vi "main.vi"() -> ()   [LabVIEW 2018]
uses:
  Interface/Interface.lvclass
  Interface/Interface.lvclass/Interface.ctl
  CCD/CCD.lvclass/CCD.ctl
  Timer/Timer.lvclass/Timer.ctl
  JSON/JSON.lvclass/JSON.ctl
  CCD/CCD.lvclass
  Timer/Timer.lvclass
  JSON/JSON.lvclass
  State Machine/State Machine.lvclass
  Cooler/Cooler.lvclass
panel:
  in  "Camera Setup":T1={"Exposure Time"=1e-05, "Readout Rate"=0, "Pre-amp gain"=0, "Initial Line"=1, "Final Line"=1024, "Final Column"=1024, "Initial Cloumn"=1, "Binning"=1, "EM Gain"=2, "EM Mode"=0, "Kinetic Series Length"=1} {"Kinetic Series Length" min=1; "EM Mode" items=["Electron Multiplying", "Conventional"]; "EM Gain" min=2 max=300; "Binning" min=1 max=2; "Initial Cloumn" min=1 max=1024; "Final Column" min=1 max=1024; "Final Line" min=1 max=1024; "Initial Line" min=1 max=1024; "Pre-amp gain" items=["Gain 1", "Gain 2"]; "Readout Rate" items=["30 MHz", "20 MHz", "10 MHz", "  1 MHz"]; "Exposure Time" min=1e-05}
  in  "Camera Setup":T2={"Image Name"="Image", "# Images"=0, "Exposure Time"=0.0, "Pre-amp gain"=0, "Readout Rate"=0, "EM Mode"=0, "EM Gain"=2, "Vertical Binning"=1, "Horizontal Binning"=1, "Initial Line"=1, "Initial Cloumn"=1, "Final Line"=1024, "Final Column"=1024, "Kinetic Serie Length"=0, "Image path"="", "Shutter Mode"=2} {"Shutter Mode" items=["Auto", "Open", "Closed"]; "EM Mode" items=["Electron Multiplying", "Conventional"]; "Readout Rate" items=["1 MHz", "10 MHz", "20 MHz", "30 MHz"]; "Pre-amp gain" items=["Gain 1", "Gain 2"]}
  out "TEMP STATUS":string
  in  "Tab Control":enum32{"Front Panel", "Setup"}(tab)
  in  "JSON File Path":path
  in  "# Images":u16=1 min=1
  in  "JSON Aqc":bool
  out "Serial Number":u16
  in  "Stop Button":bool
  in  "Night Directory":string="C:\\Users\\observer\\Desktop\\Imagens_CCD\\EXP1\\"
  out "Exposições realizadas":u8(slide) max=1 scale=0.0..1.0
  out "Initialization":bool
  out "% Acquired":dbl format="%#.2g"
  out "Temperature":i16=20
  in  "Image Name":string="img"
  out "Exposing":bool
  in  "Abort":bool
  in  "Adquirir":bool
  in  "Stop Acq":bool
  in  "Pausar":bool
  in  "Shutter Mode":u16(ring)=2 items=["Auto", "Open", "Closed"]
  in  "Kinetic Series Length":u16=1 min=1
  in  "EM Mode":u8(ring) items=["Electron Multiplying", "Conventional"]
  in  "EM Gain":u32=2 min=2 max=300
  in  "Binning":u8=1 min=1 max=2
  in  "Initial Cloumn":u16=1 min=1 max=1024
  in  "Final Column":u16=1024 min=1 max=1024
  in  "Final Line":u16=1024 min=1 max=1024
  in  "Initial Line":u16=1 min=1 max=1024
  in  "Sub Image":T3(radio)=enum."1024 x 1024"
  in  "Pre-amp gain":u8(ring) items=["Gain 1", "Gain 2"]
  in  "Readout Rate":u8(ring) items=["   1 MHz", "0.1 MHz"]
  in  "Exposure Time":dbl=1e-05 min=1e-05
  in  "Set temperature":i16=20 min=-80 max=20
  in  "Cooler ON/OFF":u16(ring) items=["Cooler OFF", "Cooler ON"]
  in  "Save Setup":bool
  in  "Load Setup":bool
  # "Macro Sparc4:\nAcquisition Controller"
  # "JSON Interface"
  # "Timings"
  # "Temperature & Shutter"
  # "HSS & Preamp"
  # "EM Mode"
  # "Sub Image & Binning"
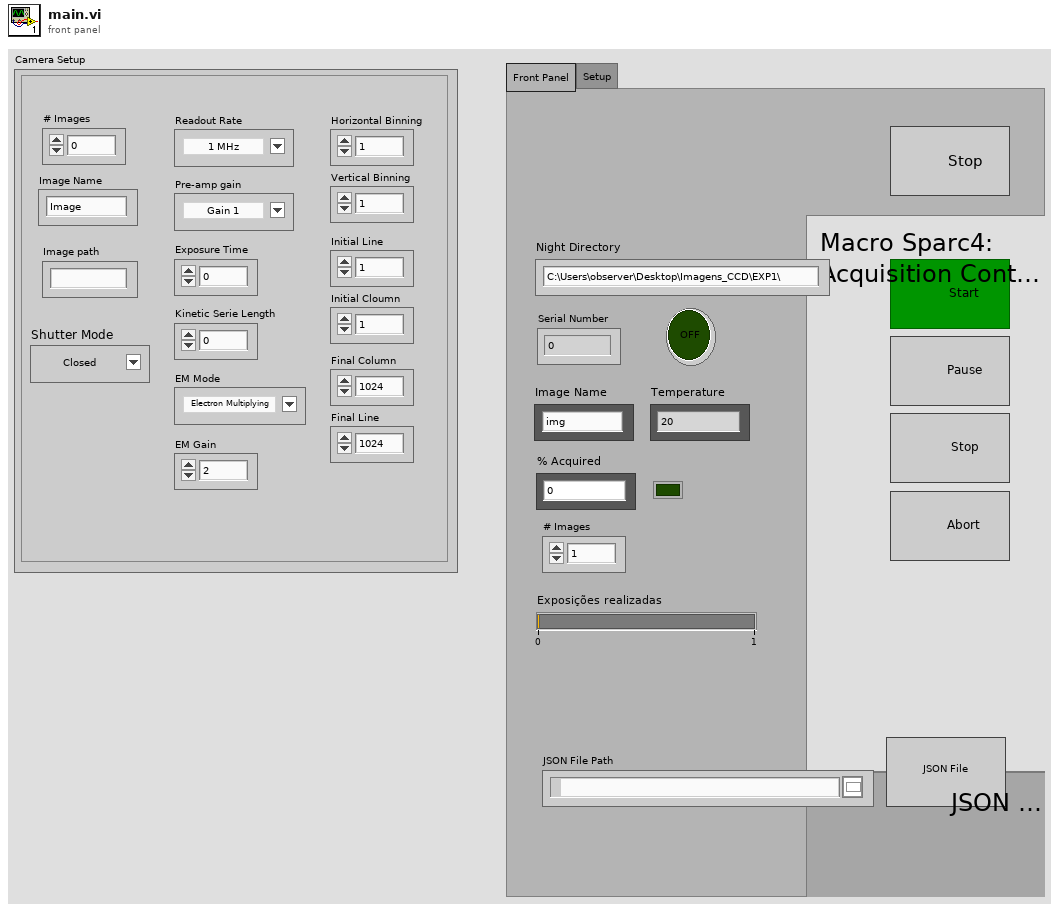
[diagram p1: front panel]
types:
  T1 = cluster{"Exposure Time":dbl, "Readout Rate":u8, "Pre-amp gain":u8, "Initial Line":u16, "Final Line":u16, "Final Column":u16, "Initial Cloumn":u16, "Binning":u8, "EM Gain":u16, "EM Mode":u8, "Kinetic Series Length":u16}
  T2 = cluster{"Image Name":string, "# Images":u32, "Exposure Time":dbl, "Pre-amp gain":u8, "Readout Rate":u8, "EM Mode":u8, "EM Gain":u32, "Vertical Binning":u16, "Horizontal Binning":u16, "Initial Line":u16, "Initial Cloumn":u16, "Final Line":u16, "Final Column":u16, "Kinetic Serie Length":u32, "Image path":string, "Shutter Mode":u16}
  T3 = enum32{"256 x 256", "512 x 512", "1024 x 1024", "Custom"}
  T4 = enum8{"Enabled", "Disabled", "Disabled and Grayed Out"}
  T5 = cluster{"Acquiring":bool, "%Acquired":dbl, "Actual Temperature":i16, "Temperature Status":string}
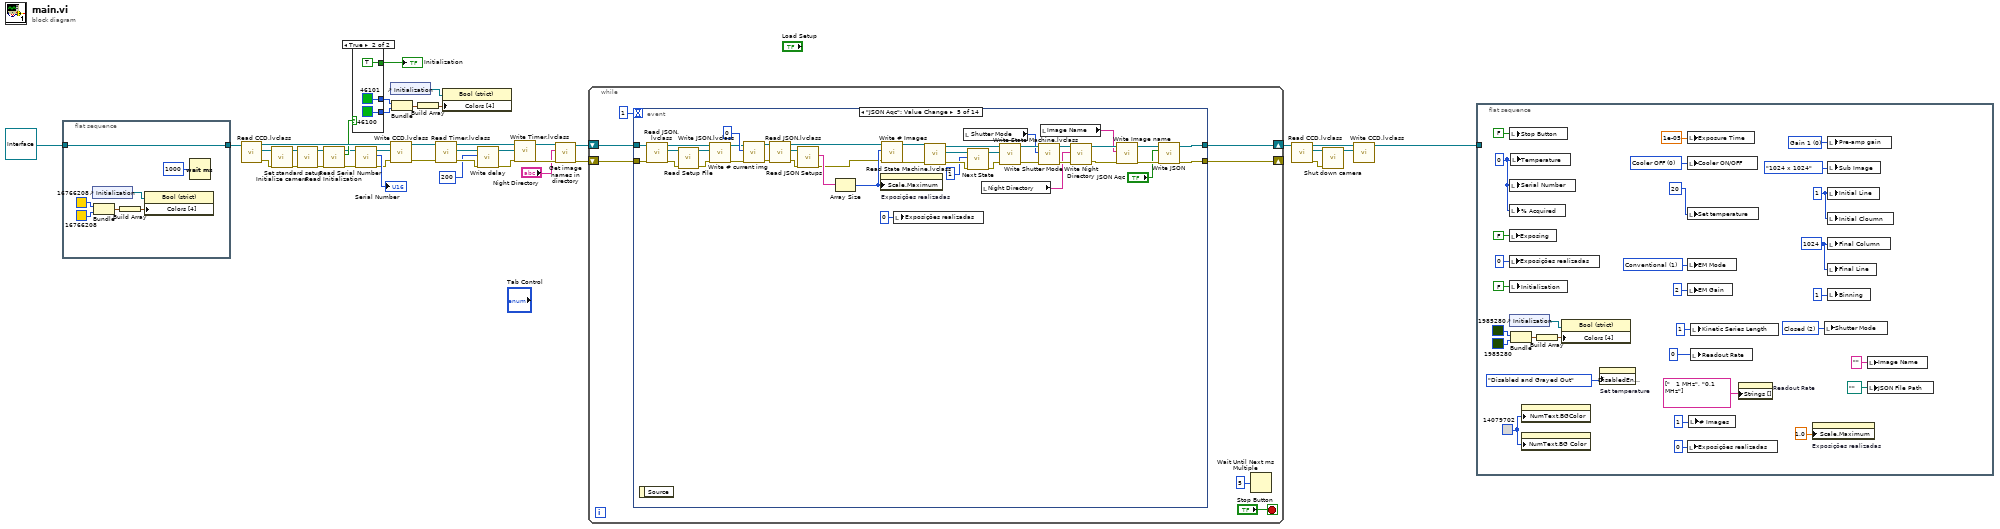
[diagram p0: block diagram]
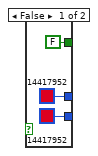
[diagram p2: hidden frame]
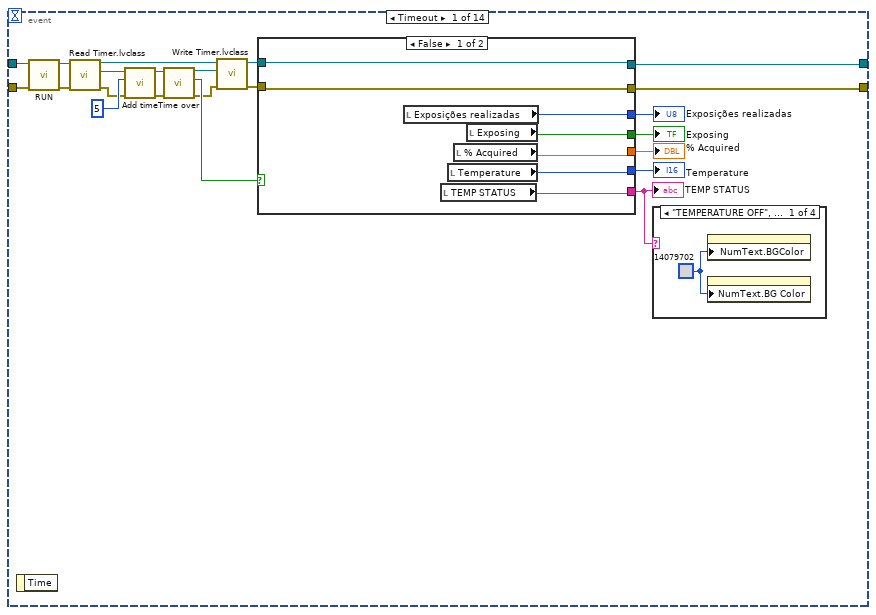
[diagram p3: hidden frame]
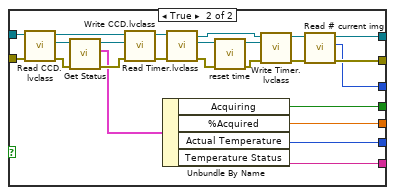
[diagram p4: hidden frame]
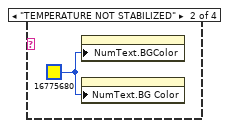
[diagram p5: hidden frame]
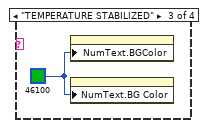
[diagram p6: hidden frame]
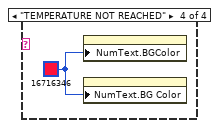
[diagram p7: hidden frame]
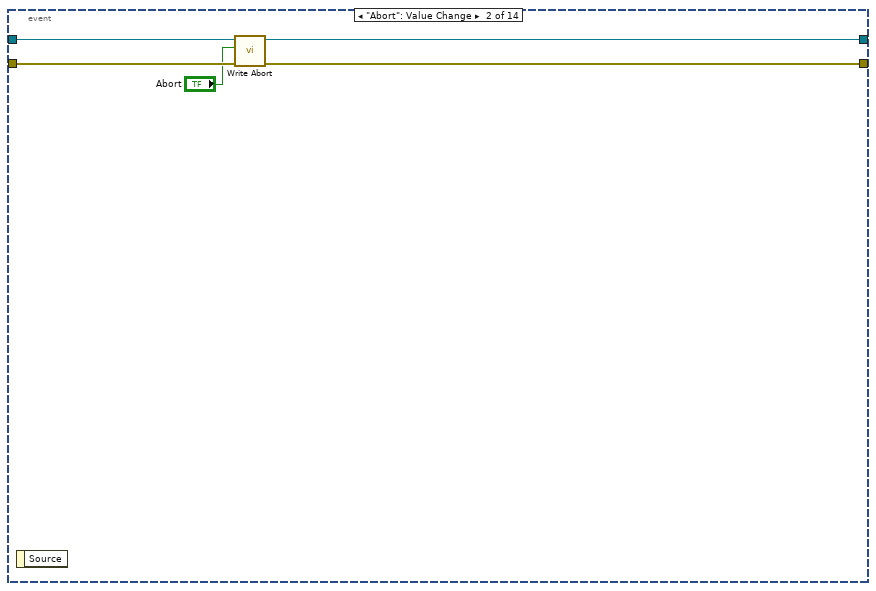
[diagram p8: hidden frame]
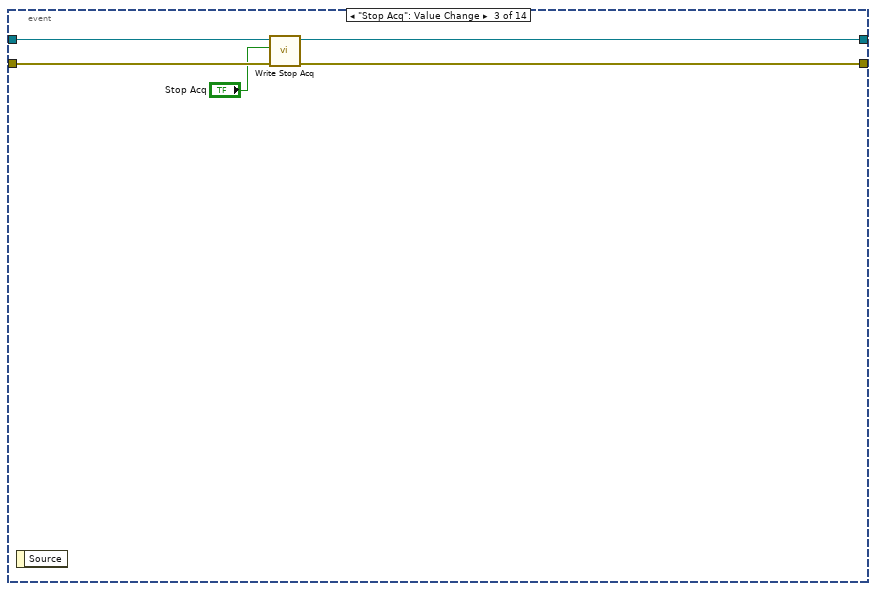
[diagram p9: hidden frame]
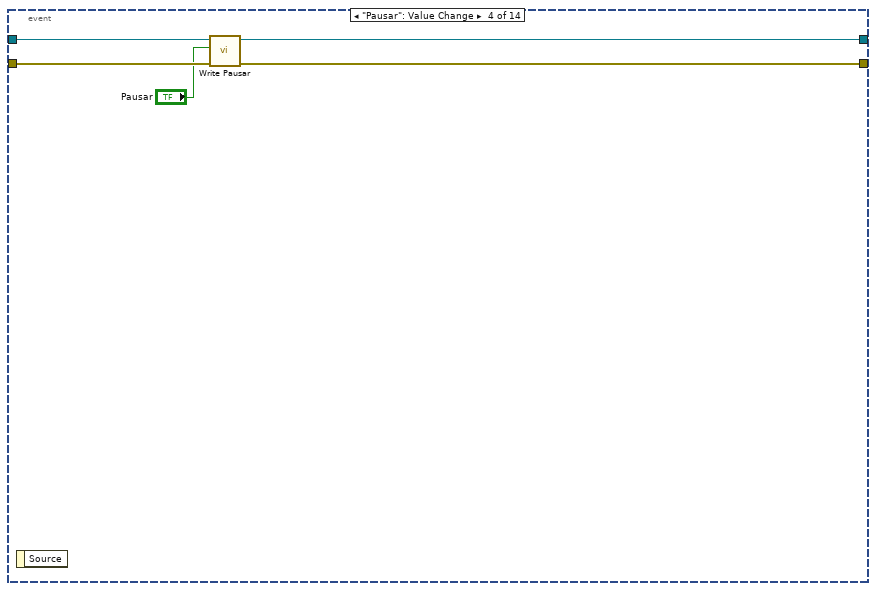
[diagram p10: hidden frame]
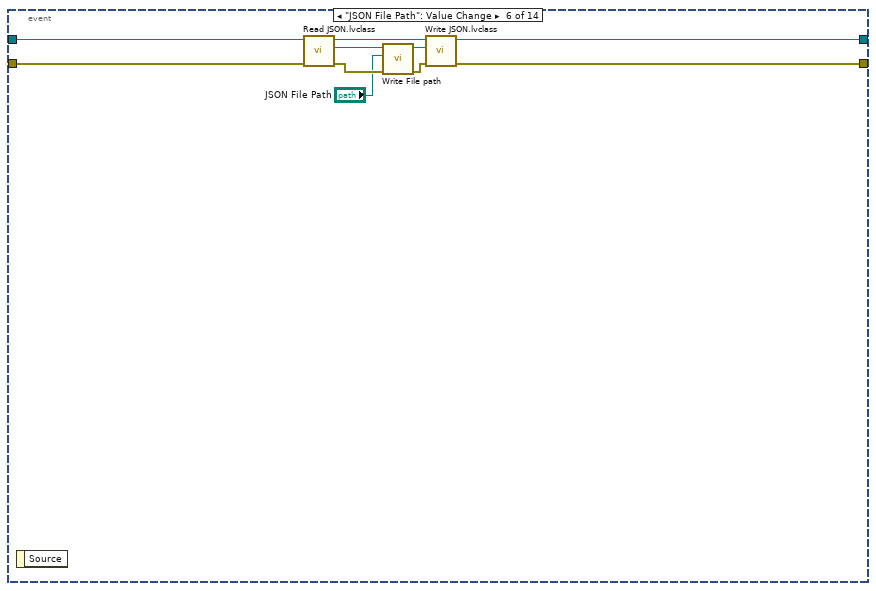
[diagram p11: hidden frame]
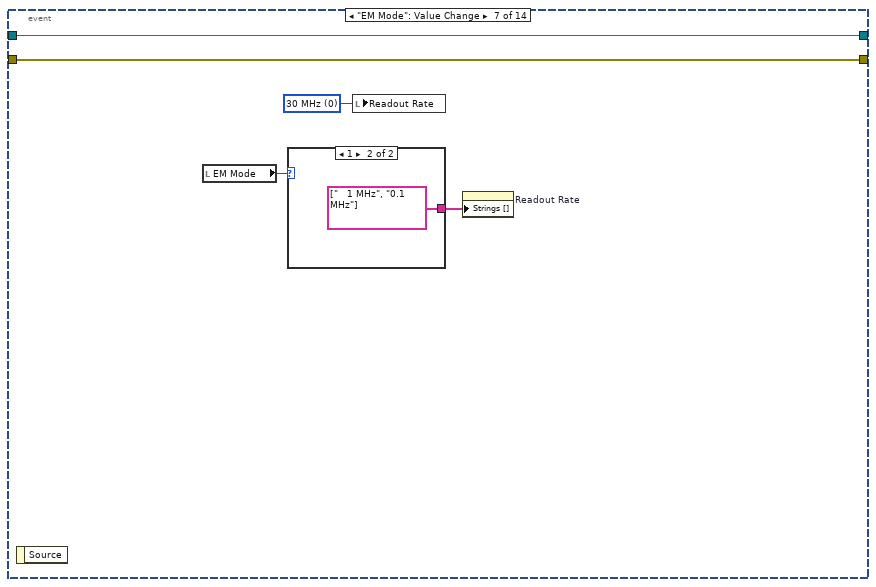
[diagram p12: hidden frame]
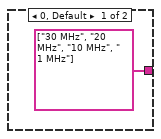
[diagram p13: hidden frame]
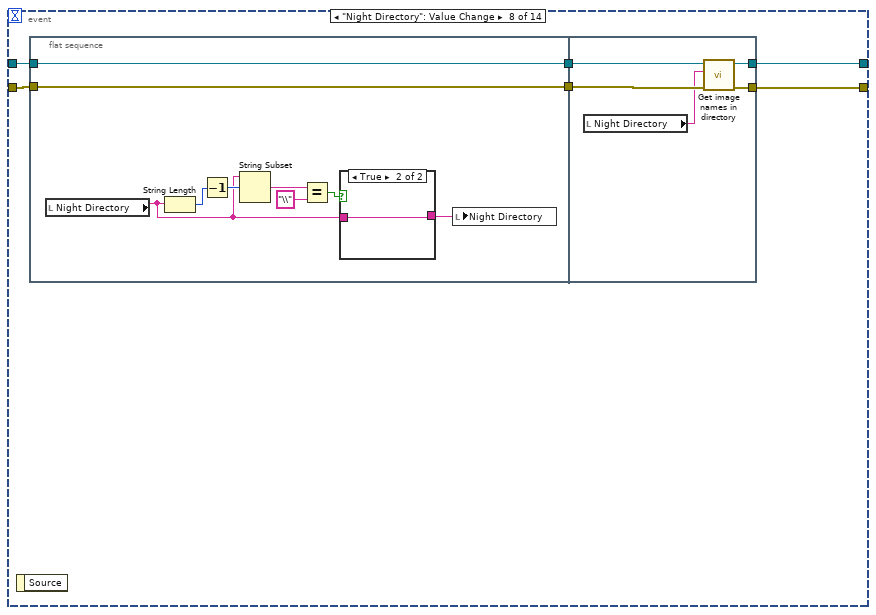
[diagram p14: hidden frame]
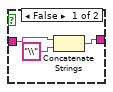
[diagram p15: hidden frame]
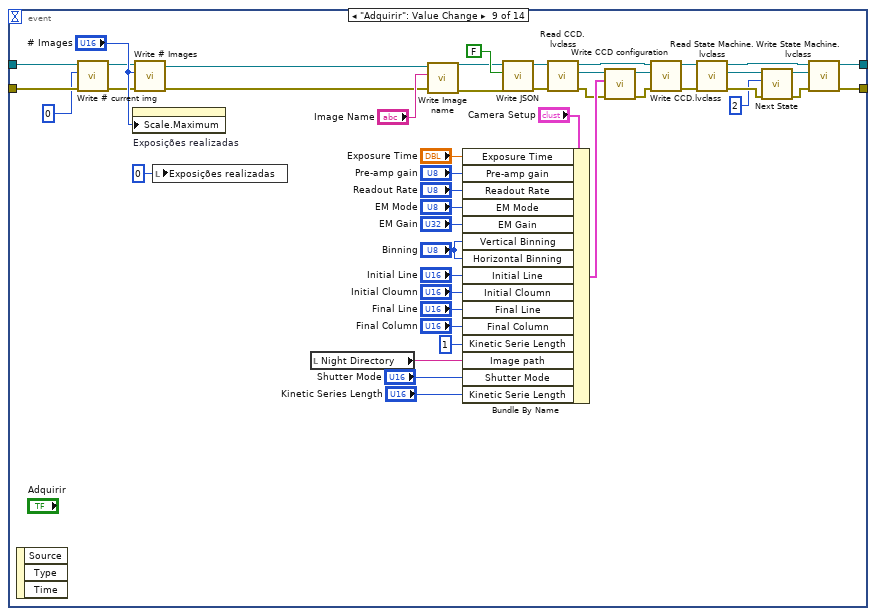
[diagram p16: hidden frame]
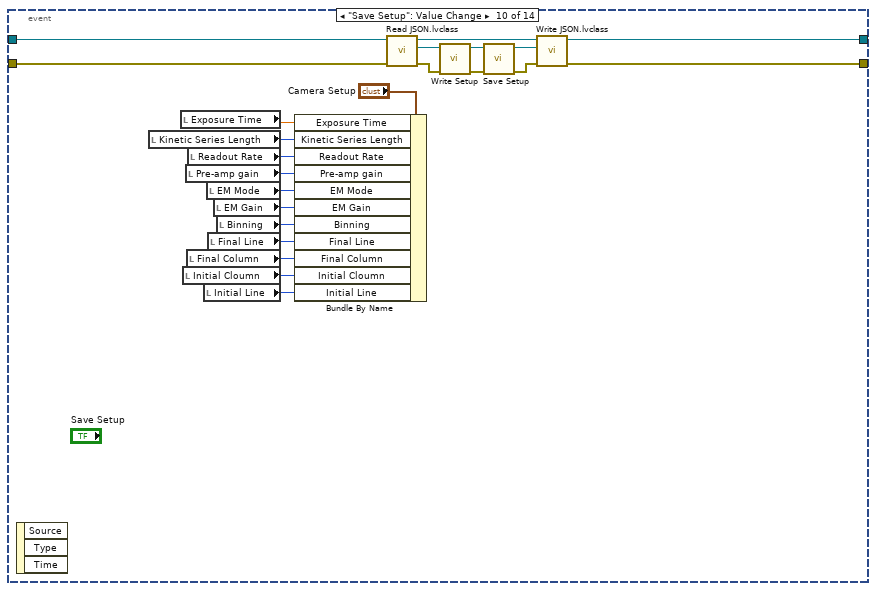
[diagram p17: hidden frame]
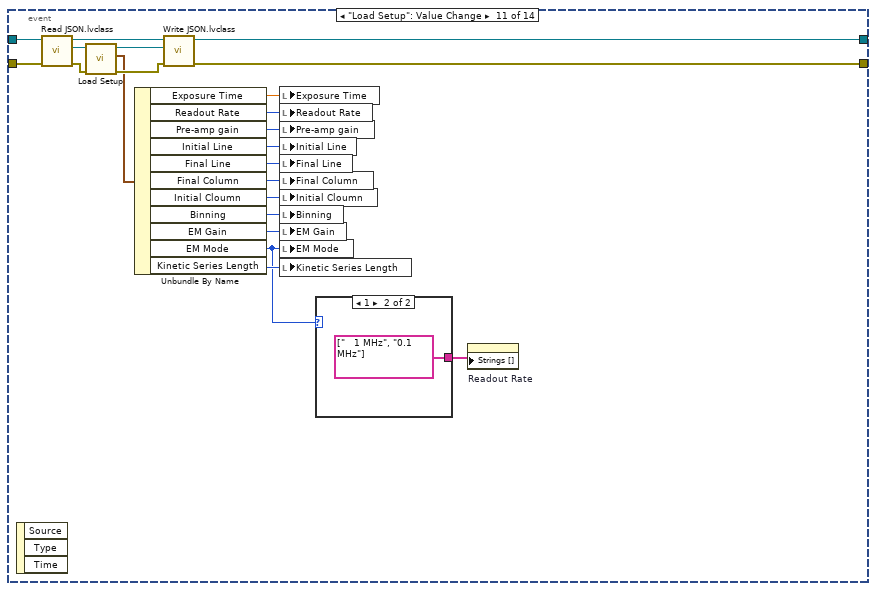
[diagram p18: hidden frame]
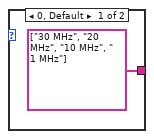
[diagram p19: hidden frame]
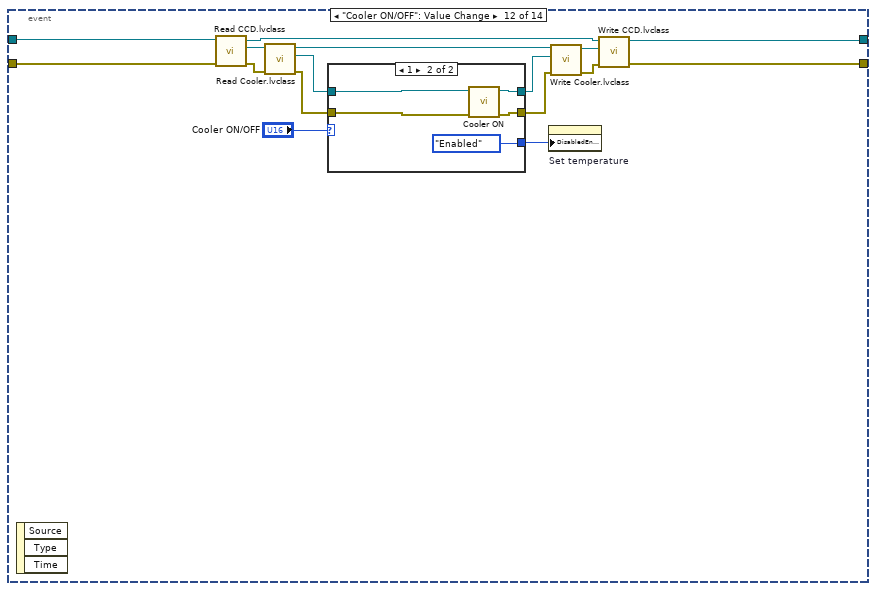
[diagram p20: hidden frame]
diagram:
  n1 = flat-sequence {
    tunnel: [w47] -> w16
    tunnel: refnum<class "Interface.lvclass"> refnum ("Interface.lvclass") -> [w47]
    frame #0 {
      n2 = control-ref of="Initialization"() -> (w46:refnum<vi>)
      n3 = Bundle(u32 16766208, u32 16766208) -> (w44:cluster{u32, u32})  [unwired: 1 in]
      n4 = Build Array(w44) -> (w45:cluster{u32, u32}[])
      n5 = property on="Property Node" class="Bool (strict)"(reference=w46, "Colors [4]"=w45) -> ()  [unwired: 1 in, 2 out]
      n6 = Wait (ms)(milliseconds to wait=u32 1000) -> ()  [unwired: 1 out]
    }
  }
  n7 = call "Read CCD.lvclass.vi"("Interface in"=w16) -> ("error out"=w38:errorcluster, "CCD.lvclass"=w40:refnum<class "CCD.lvclass">, "Interface out"=w37:refnum<class "Interface.lvclass">)  [unwired: 8 in]
  n8 = call "Initialize camera.vi"("error in (no error)"=w38, "CCD in"=w40) -> ("error out"=w36:errorcluster, "CCD out"=w39:refnum<class "CCD.lvclass">)  [unwired: 8 in]
  n9 = call "Set standard setup.vi"("error in (no error)"=w36, "CCD in"=w39) -> ("error out"=w29:errorcluster, "CCD out"=w30:refnum<class "CCD.lvclass">)  [unwired: 8 in]
  n10 = call "Read Initialization.vi"("error in (no error)"=w29, "CCD in"=w30) -> ("error out"=w22:errorcluster, "Initialization"=w28:bool, "CCD out"=w21:refnum<class "CCD.lvclass">)  [unwired: 7 in]
  n11 = case shown="True" w28 {
    tunnel: [u32 14417952 u32 46100] -> w24
    tunnel: [u32 14417952 u32 46101] -> w23
    tunnel: [FALSE TRUE] -> w1
    frame False {
    }
    frame True {
    }
  }
  "Initialization" <- w1
  n12 = call "Read Serial Number.vi"("error in (no error)"=w22, "CCD in"=w21) -> ("error out"=w19:errorcluster, "Serial Number"=→"Serial Number":u32, "CCD out"=w18:refnum<class "CCD.lvclass">)  [unwired: 7 in]
  n13 = control-ref of="Initialization"() -> (w27:refnum<vi>)
  n14 = call "Write CCD.lvclass.vi"("error in (no error)"=w19, "CCD.lvclass"=w18, "Interface in"=w37) -> ("error out"=w15:errorcluster, "Interface out"=w14:refnum<class "Interface.lvclass">)  [unwired: 7 in]
  n15 = Bundle(w23, w24) -> (w25:cluster{u32, u32})  [unwired: 1 in]
  n16 = Build Array(w25) -> (w26:cluster{u32, u32}[])
  n17 = call "Read Timer.lvclass.vi"("error in (no error)"=w15, "Interface in"=w14) -> ("error out"=w9:errorcluster, "Timer.lvclass"=w13:refnum<class "Timer.lvclass">, "Interface out"=w11:refnum<class "Interface.lvclass">)  [unwired: 7 in]
  n18 = property on="Property Node" class="Bool (strict)"(reference=w27, "Colors [4]"=w26) -> ()  [unwired: 1 in, 2 out]
  n19 = call "Write delay.vi"("error in (no error)"=w9, "delay"=u32 200, "Timer in"=w13) -> ("error out"=w10:errorcluster, "Timer out"=w12:refnum<class "Timer.lvclass">)  [unwired: 7 in]
  n20 = call "Write Timer.lvclass.vi"("error in (no error)"=w10, "Timer.lvclass"=w12, "Interface in"=w11) -> ("error out"=w3:errorcluster, "Interface out"=w4:refnum<class "Interface.lvclass">)  [unwired: 7 in]
  n21 = call "Get image names in directory.vi"("error in (no error)"=w3, "Image Path"="Night Directory", "Interface in"=w4) -> ("error out"=w6:errorcluster, "Interface out"=w5:refnum<class "Interface.lvclass">)  [unwired: 7 in]
  n22 = while {
    shift-right: [w56] -> w35
    shift-left: w5 -> [w57]
    shift-right: [w55] -> _
    shift-left: w6 -> [w54]
    stop <- "Stop Button" stop-if-true
    n23 = event shown="[4] \"JSON Aqc\": Value Change" {
      selector: _ -> [_ _ _ _ _ _ _ _ _ _ _ _ _ _]
      dyn-events: _ -> [_ _ _ _ _ _ _ _ _ _ _ _ _ _]
      timeout: 1 -> [_ _ _ _ _ _ _ _ _ _ _ _ _ _]
      tunnel: w57 -> [w82 w122 w127 w132 w173 w183 w188 w195 w225 w283 w304 w322 w339 w369]
      tunnel: [w63 w120 w125 w130 w135 w180 w188 w192 w235 w280 w302 w321 w339 w360] -> w56
      tunnel: [w62 w119 w124 w129 w134 w179 w187 w191 w234 w279 w301 w320 w334 w359] -> w55
      tunnel: w54 -> [w81 w121 w126 w131 w172 w182 w187 w193 w224 w282 w303 w323 w334 w368]
      event Timeout {
        n24 = event-data() -> ()  [unwired: 1 in, 1 out]
        n25 = call "RUN.vi"("error in (no error)"=w81, "Interface in"=w82) -> ("error out"=w77:errorcluster, "Interface out"=w76:refnum<class "Interface.lvclass">)  [unwired: 8 in]
        n26 = call "Read Timer.lvclass.vi"("error in (no error)"=w77, "Interface in"=w76) -> ("error out"=w73:errorcluster, "Timer.lvclass"=w75:refnum<class "Timer.lvclass">, "Interface out"=w70:refnum<class "Interface.lvclass">)  [unwired: 7 in]
        n27 = call "Add time.vi"("error in (no error)"=w73, "Numeric Control"=u32 5, "Timer in"=w75) -> ("error out"=w72:errorcluster, "Timer out"=w71:refnum<class "Timer.lvclass">)  [unwired: 7 in]
        n28 = call "Time over.vi"("error in (no error)"=w72, "Timer in"=w71) -> ("error out"=w67:errorcluster, "time over"=w69:bool, "Timer out"=w66:refnum<class "Timer.lvclass">)  [unwired: 7 in]
        n29 = call "Write Timer.lvclass.vi"("error in (no error)"=w67, "Timer.lvclass"=w66, "Interface in"=w70) -> ("error out"=w65:errorcluster, "Interface out"=w64:refnum<class "Interface.lvclass">)  [unwired: 7 in]
        n30 = case shown="False" w69 {
          tunnel: [w87 w113] -> w80
          tunnel: [w88 w112] -> w79
          tunnel: [w89 w111] -> w78
          tunnel: [w86 w110] -> w68
          tunnel: w65 -> [w84 w103]
          tunnel: w64 -> [w85 w102]
          tunnel: [w85 w92] -> w63
          tunnel: [w84 w91] -> w62
          tunnel: [w83 w90] -> w61
          frame False {
            n31 = local read "Exposições realizadas"() -> (w83:u8)
            n32 = local read "TEMP STATUS"() -> (w86:string)
            n33 = local read "Temperature"() -> (w89:i16)
            n34 = local read "% Acquired"() -> (w88:dbl)
            n35 = local read "Exposing"() -> (w87:bool)
          }
          frame True {
            n36 = call "Read CCD.lvclass.vi"("error in (no error)"=w103, "Interface in"=w102) -> ("error out"=w107:errorcluster, "CCD.lvclass"=w106:refnum<class "CCD.lvclass">, "Interface out"=w105:refnum<class "Interface.lvclass">)  [unwired: 7 in]
            n37 = call "Get Status.vi"("error in (no error)"=w107, "CCD in"=w106) -> ("error out"=w109:errorcluster, "Camera Status"=w104:T5, "CCD out"=w108:refnum<class "CCD.lvclass">)  [unwired: 7 in]
            n38 = call "Write CCD.lvclass.vi"("error in (no error)"=w109, "CCD.lvclass"=w108, "Interface in"=w105) -> ("error out"=w101:errorcluster, "Interface out"=w100:refnum<class "Interface.lvclass">)  [unwired: 7 in]
            n39 = Unbundle By Name(w104) -> ("Acquiring"=w113:bool, "%Acquired"=w112:dbl, "Actual Temperature"=w111:i16, "Temperature Status"=w110:string)
            n40 = call "Read Timer.lvclass.vi"("error in (no error)"=w101, "Interface in"=w100) -> ("error out"=w98:errorcluster, "Timer.lvclass"=w99:refnum<class "Timer.lvclass">, "Interface out"=w96:refnum<class "Interface.lvclass">)  [unwired: 7 in]
            n41 = call "reset time.vi"("error in (no error)"=w98, "Timer in"=w99) -> ("error out"=w95:errorcluster, "Timer out"=w97:refnum<class "Timer.lvclass">)  [unwired: 8 in]
            n42 = call "Write Timer.lvclass.vi"("error in (no error)"=w95, "Timer.lvclass"=w97, "Interface in"=w96) -> ("error out"=w94:errorcluster, "Interface out"=w93:refnum<class "Interface.lvclass">)  [unwired: 7 in]
            n43 = call "Read # current img.vi"("error in (no error)"=w94, "Interface in"=w93) -> ("error out"=w91:errorcluster, "# current img"=w90:u16, "Interface out"=w92:refnum<class "Interface.lvclass">)  [unwired: 7 in]
          }
        }
        "Exposing" <- w80
        "% Acquired" <- w79
        "Temperature" <- w78
        "TEMP STATUS" <- w68
        "Exposições realizadas" <- w61
        n44 = case shown="\"TEMPERATURE OFF\", Default" w68 {
          frame "TEMPERATURE OFF", Default {
            w114 = u32 14079702
            n45 = property on="Temperature" class="DigNum (strict)"("NumText.BGColor"=w114) -> ()  [unwired: 2 in, 2 out]
            n46 = property on="Temperature" class="DigNum (strict)"("NumText.BG Color"=w114) -> ()  [unwired: 2 in, 2 out]
          }
          frame "TEMPERATURE NOT STABILIZED" {
            w115 = u32 16775680
            n47 = property on="Temperature" class="DigNum (strict)"("NumText.BGColor"=w115) -> ()  [unwired: 2 in, 2 out]
            n48 = property on="Temperature" class="DigNum (strict)"("NumText.BG Color"=w115) -> ()  [unwired: 2 in, 2 out]
          }
          frame "TEMPERATURE STABILIZED" {
            w116 = u32 46100
            n49 = property on="Temperature" class="DigNum (strict)"("NumText.BGColor"=w116) -> ()  [unwired: 2 in, 2 out]
            n50 = property on="Temperature" class="DigNum (strict)"("NumText.BG Color"=w116) -> ()  [unwired: 2 in, 2 out]
          }
          frame "TEMPERATURE NOT REACHED" {
            w117 = u32 16716346
            n51 = property on="Temperature" class="DigNum (strict)"("NumText.BGColor"=w117) -> ()  [unwired: 2 in, 2 out]
            n52 = property on="Temperature" class="DigNum (strict)"("NumText.BG Color"=w117) -> ()  [unwired: 2 in, 2 out]
          }
        }
      }
      event "Abort": Value Change {
        n53 = event-data() -> ()  [unwired: 1 in, 1 out]
        n54 = call "Write Abort.vi"("error in (no error)"=w121, "Abort"="Abort", "Interface in"=w122) -> ("error out"=w119:errorcluster, "Interface out"=w120:refnum<class "Interface.lvclass">)  [unwired: 7 in]
      }
      event "Stop Acq": Value Change {
        n55 = event-data() -> ()  [unwired: 1 in, 1 out]
        n56 = call "Write Stop Acq.vi"("error in (no error)"=w126, "Stop Acq"="Stop Acq", "Interface in"=w127) -> ("error out"=w124:errorcluster, "Interface out"=w125:refnum<class "Interface.lvclass">)  [unwired: 7 in]
      }
      event "Pausar": Value Change {
        n57 = event-data() -> ()  [unwired: 1 in, 1 out]
        n58 = call "Write Pausar.vi"("error in (no error)"=w131, "Pausar"="Pausar", "Interface in"=w132) -> ("error out"=w129:errorcluster, "Interface out"=w130:refnum<class "Interface.lvclass">)  [unwired: 7 in]
      }
      event "JSON Aqc": Value Change {
        n59 = event-data() -> ()  [unwired: 1 in, 1 out]
        n60 = call "Read JSON.lvclass.vi"("error in (no error)"=w172, "Interface in"=w173) -> ("error out"=w167:errorcluster, "JSON.lvclass"=w168:refnum<class "JSON.lvclass">, "Interface out"=w171:refnum<class "Interface.lvclass">)  [unwired: 7 in]
        n61 = call "Read Setup File.vi"("error in (no error)"=w167, "JSON in"=w168) -> ("error out"=w169:errorcluster, "JSON out"=w170:refnum<class "JSON.lvclass">)  [unwired: 8 in]
        n62 = call "Write JSON.lvclass.vi"("error in (no error)"=w169, "JSON.lvclass"=w170, "Interface in"=w171) -> ("error out"=w147:errorcluster, "Interface out"=w148:refnum<class "Interface.lvclass">)  [unwired: 7 in]
        n63 = call "Write # current img.vi"("error in (no error)"=w147, "# current img"=0, "Interface in"=w148) -> ("error out"=w156:errorcluster, "Interface out"=w155:refnum<class "Interface.lvclass">)  [unwired: 7 in]
        n64 = call "Read JSON.lvclass.vi"("error in (no error)"=w156, "Interface in"=w155) -> ("error out"=w153:errorcluster, "JSON.lvclass"=w154:refnum<class "JSON.lvclass">, "Interface out"=w150:refnum<class "Interface.lvclass">)  [unwired: 7 in]
        n65 = call "Read JSON Setups.vi"("error in (no error)"=w153, "JSON in"=w154) -> ("error out"=w149:errorcluster, "JSON Setups"=w152:string[])  [unwired: 7 in, 1 out]
        n66 = Array Size(array=w152) -> (size(s)=w151:i32)
        n67 = property on="Exposições realizadas" class="Slide (strict)"("Scale.Maximum"=w151) -> ()  [unwired: 2 in, 2 out]
        n68 = call "Write # Images.vi"("error in (no error)"=w149, "# Images"=w151, "Interface in"=w150) -> ("error out"=w157:errorcluster, "Interface out"=w158:refnum<class "Interface.lvclass">)  [unwired: 7 in]
        n69 = local write "Exposições realizadas"(u8 0 ("Exposições realizadas")) -> ()
        n70 = call "Read State Machine.lvclass.vi"("error in (no error)"=w157, "Interface in"=w158) -> ("error out"=w165:errorcluster, "State Machine.lvclass"=w166:refnum<class "State Machine.lvclass">, "Interface out"=w162:refnum<class "Interface.lvclass">)  [unwired: 7 in]
        n71 = local read "Shutter Mode"() -> (w141:u16)
        n72 = call "Next State.vi"("error in (no error)"=w165, "New_State"=1, "State Machine in"=w166) -> ("error out"=w164:errorcluster, "State Machine out"=w163:refnum<class "State Machine.lvclass">)  [unwired: 7 in]
        n73 = local read "Night Directory"() -> (w142:string)
        n74 = call "Write State Machine.lvclass.vi"("error in (no error)"=w164, "State Machine.lvclass"=w163, "Interface in"=w162) -> ("error out"=w145:errorcluster, "Interface out"=w146:refnum<class "Interface.lvclass">)  [unwired: 7 in]
        n75 = call "Write Shutter Mode.vi"("error in (no error)"=w145, "Shutter Mode"=w141, "Interface in"=w146) -> ("error out"=w143:errorcluster, "Interface out"=w144:refnum<class "Interface.lvclass">)  [unwired: 7 in]
        n76 = local read "Image Name"() -> (w138:string)
        n77 = call "Write Night Directory.vi"("error in (no error)"=w143, "Night Directory"=w142, "Interface in"=w144) -> ("error out"=w139:errorcluster, "Interface out"=w140:refnum<class "Interface.lvclass">)  [unwired: 7 in]
        n78 = call "Write Image name.vi"("error in (no error)"=w139, "Image name"=w138, "Interface in"=w140) -> ("error out"=w137:errorcluster, "Interface out"=w136:refnum<class "Interface.lvclass">)  [unwired: 7 in]
        n79 = call "Write JSON.vi"("error in (no error)"=w137, "JSON"="JSON Aqc", "Interface in"=w136) -> ("error out"=w134:errorcluster, "Interface out"=w135:refnum<class "Interface.lvclass">)  [unwired: 7 in]
      }
      event "JSON File Path": Value Change {
        n80 = event-data() -> ()  [unwired: 1 in, 1 out]
        n81 = call "Read JSON.lvclass.vi"("error in (no error)"=w182, "Interface in"=w183) -> ("error out"=w175:errorcluster, "JSON.lvclass"=w178:refnum<class "JSON.lvclass">, "Interface out"=w181:refnum<class "Interface.lvclass">)  [unwired: 7 in]
        n82 = call "Write File path.vi"("error in (no error)"=w175, "File path"="JSON File Path", "JSON in"=w178) -> ("error out"=w176:errorcluster, "JSON out"=w177:refnum<class "JSON.lvclass">)  [unwired: 7 in]
        n83 = call "Write JSON.lvclass.vi"("error in (no error)"=w176, "JSON.lvclass"=w177, "Interface in"=w181) -> ("error out"=w179:errorcluster, "Interface out"=w180:refnum<class "Interface.lvclass">)  [unwired: 7 in]
      }
      event "EM Mode": Value Change {
        w185 = u8 0 items=["30 MHz", "20 MHz", "10 MHz", "1 MHz"] ("Readout Rate")
        n84 = event-data() -> ()  [unwired: 1 in, 1 out]
        n85 = local read "EM Mode"() -> (w186:u8)
        n86 = case shown="1" w186 {
          tunnel: [string[] ["30 MHz", "20 MHz", "10 MHz", "  1 MHz"] string[] ["   1 MHz", "0.1 MHz"]] -> w184
          frame 0, Default {
          }
          frame 1 {
          }
        }
        n87 = local write "Readout Rate"(w185) -> ()
        n88 = property on="Readout Rate" class="Ring (strict)"("Strings []"=w184) -> ()  [unwired: 2 in, 2 out]
      }
      event "Night Directory": Value Change {
        n89 = event-data() -> ()  [unwired: 1 in, 1 out]
        n90 = flat-sequence {
          tunnel: [w198] -> w196
          tunnel: w195 -> [w198]
          tunnel: [w197] -> w194
          tunnel: w193 -> [w197]
          tunnel: w196 -> [w213]
          tunnel: w194 -> [w214]
          tunnel: [w212] -> w192
          tunnel: [w211] -> w191
          frame #0 {
            n91 = local read "Night Directory"() -> (w201:string)
            n92 = String Length(string=w201) -> (length=w205:i32)
            n93 = Decrement(x=w205) -> (x-1=w204:i32)
            n94 = String Subset(string=w201, offset (0)=w204) -> (substring=w203:string)  [unwired: 1 in]
            n95 = Equal?(x=w203, y="\\") -> (x = y?=w202:bool)
            n96 = case shown="True" w202 {
              tunnel: [w208 w209] -> w200
              tunnel: w201 -> [w206 w209]
              frame False {
                n97 = Concatenate Strings(w206, "\\") -> (w208:string)
              }
              frame True {
              }
            }
            n98 = local write "Night Directory"(w200) -> ()
          }
          frame #1 {
            n99 = local read "Night Directory"() -> (w210:string)
            n100 = call "Get image names in directory.vi"("error in (no error)"=w214, "Image Path"=w210, "Interface in"=w213) -> ("error out"=w211:errorcluster, "Interface out"=w212:refnum<class "Interface.lvclass">)  [unwired: 7 in]
          }
        }
      }
      event "Adquirir": Value Change {
        n101 = event-data() -> ()  [unwired: 1 in, 3 out]
        n102 = call "Write # current img.vi"("error in (no error)"=w224, "# current img"=0, "Interface in"=w225) -> ("error out"=w227:errorcluster, "Interface out"=w226:refnum<class "Interface.lvclass">)  [unwired: 7 in]
        n103 = property on="Exposições realizadas" class="Slide (strict)"("Scale.Maximum"="# Images") -> ()  [unwired: 2 in, 2 out]
        n104 = call "Write # Images.vi"("error in (no error)"=w227, "# Images"="# Images", "Interface in"=w226) -> ("error out"=w215:errorcluster, "Interface out"=w216:refnum<class "Interface.lvclass">)  [unwired: 7 in]
        n105 = local write "Exposições realizadas"(u8 0 ("Exposições realizadas")) -> ()
        n106 = local read "Night Directory"() -> (w233:string)
        n107 = call "Write Image name.vi"("error in (no error)"=w215, "Image name"="Image Name", "Interface in"=w216) -> ("error out"=w218:errorcluster, "Interface out"=w217:refnum<class "Interface.lvclass">)  [unwired: 7 in]
        n108 = Bundle By Name(cluster="Camera Setup", "Exposure Time"="Exposure Time", "Pre-amp gain"="Pre-amp gain", "Readout Rate"="Readout Rate", "EM Mode"="EM Mode", "EM Gain"="EM Gain", "Vertical Binning"="Binning", "Horizontal Binning"="Binning", "Initial Line"="Initial Line", "Initial Cloumn"="Initial Cloumn", "Final Line"="Final Line", "Final Column"="Final Column", "Kinetic Serie Length"=u32 1, "Image path"=w233, "Shutter Mode"="Shutter Mode", "Kinetic Serie Length"="Kinetic Series Length") -> (w248:T2)
        n109 = call "Write JSON.vi"("error in (no error)"=w218, "JSON"=FALSE, "Interface in"=w217) -> ("error out"=w222:errorcluster, "Interface out"=w221:refnum<class "Interface.lvclass">)  [unwired: 7 in]
        n110 = call "Read CCD.lvclass.vi"("error in (no error)"=w222, "Interface in"=w221) -> ("error out"=w246:errorcluster, "CCD.lvclass"=w247:refnum<class "CCD.lvclass">, "Interface out"=w244:refnum<class "Interface.lvclass">)  [unwired: 7 in]
        n111 = call "Write CCD configuration.vi"("error in (no error)"=w246, "Camera Setup"=w248, "CCD in"=w247) -> ("error out"=w245:errorcluster, "CCD out"=w230:refnum<class "CCD.lvclass">)  [unwired: 7 in]
        n112 = call "Write CCD.lvclass.vi"("error in (no error)"=w245, "CCD.lvclass"=w230, "Interface in"=w244) -> ("error out"=w243:errorcluster, "Interface out"=w242:refnum<class "Interface.lvclass">)  [unwired: 7 in]
        n113 = call "Read State Machine.lvclass.vi"("error in (no error)"=w243, "Interface in"=w242) -> ("error out"=w240:errorcluster, "State Machine.lvclass"=w241:refnum<class "State Machine.lvclass">, "Interface out"=w237:refnum<class "Interface.lvclass">)  [unwired: 7 in]
        n114 = call "Next State.vi"("error in (no error)"=w240, "New_State"=2, "State Machine in"=w241) -> ("error out"=w239:errorcluster, "State Machine out"=w238:refnum<class "State Machine.lvclass">)  [unwired: 7 in]
        n115 = call "Write State Machine.lvclass.vi"("error in (no error)"=w239, "State Machine.lvclass"=w238, "Interface in"=w237) -> ("error out"=w234:errorcluster, "Interface out"=w235:refnum<class "Interface.lvclass">)  [unwired: 7 in]
      }
      event "Save Setup": Value Change {
        n116 = event-data() -> ()  [unwired: 1 in, 3 out]
        n117 = local read "Kinetic Series Length"() -> (w270:u16)
        n118 = local read "Exposure Time"() -> (w271:dbl)
        n119 = local read "Initial Cloumn"() -> (w262:u16)
        n120 = local read "Pre-amp gain"() -> (w268:u8)
        n121 = local read "Final Column"() -> (w263:u16)
        n122 = local read "Readout Rate"() -> (w269:u8)
        n123 = local read "Initial Line"() -> (w261:u16)
        n124 = local read "EM Mode"() -> (w267:u8)
        n125 = local read "Final Line"() -> (w264:u16)
        n126 = local read "EM Gain"() -> (w266:u32)
        n127 = local read "Binning"() -> (w265:u8)
        n128 = Bundle By Name(cluster="Camera Setup", "Exposure Time"=w271, "Kinetic Series Length"=w270, "Readout Rate"=w269, "Pre-amp gain"=w268, "EM Mode"=w267, "EM Gain"=w266, "Binning"=w265, "Final Line"=w264, "Final Column"=w263, "Initial Cloumn"=w262, "Initial Line"=w261) -> ()  [unwired: 1 out]
        n129 = call "Read JSON.lvclass.vi"("error in (no error)"=w282, "Interface in"=w283) -> ("error out"=w273:errorcluster, "JSON.lvclass"=w278:refnum<class "JSON.lvclass">, "Interface out"=w281:refnum<class "Interface.lvclass">)  [unwired: 7 in]
        n130 = call "Write Setup.vi"("error in (no error)"=w273, "JSON in"=w278) -> ("error out"=w274:errorcluster, "JSON out"=w277:refnum<class "JSON.lvclass">)  [unwired: 8 in]
        n131 = call "Save Setup.vi"("error in (no error)"=w274, "JSON in"=w277) -> ("error out"=w275:errorcluster, "JSON out"=w276:refnum<class "JSON.lvclass">)  [unwired: 8 in]
        n132 = call "Write JSON.lvclass.vi"("error in (no error)"=w275, "JSON.lvclass"=w276, "Interface in"=w281) -> ("error out"=w279:errorcluster, "Interface out"=w280:refnum<class "Interface.lvclass">)  [unwired: 7 in]
      }
      event "Load Setup": Value Change {
        n133 = event-data() -> ()  [unwired: 1 in, 3 out]
        n134 = call "Read JSON.lvclass.vi"("error in (no error)"=w303, "Interface in"=w304) -> ("error out"=w299:errorcluster, "JSON.lvclass"=w300:refnum<class "JSON.lvclass">, "Interface out"=w305:refnum<class "Interface.lvclass">)  [unwired: 7 in]
        n135 = call "Load Setup.vi"("error in (no error)"=w299, "JSON in"=w300) -> ("error out"=w297:errorcluster, "Camera Setup"=w296:T1, "JSON out"=w298:refnum<class "JSON.lvclass">)  [unwired: 7 in]
        n136 = Unbundle By Name(w296) -> ("Exposure Time"=w295:dbl, "Readout Rate"=w294:u8, "Pre-amp gain"=w293:u8, "Initial Line"=w292:u16, "Final Line"=w291:u16, "Final Column"=w290:u16, "Initial Cloumn"=w289:u16, "Binning"=w288:u8, "EM Gain"=w287:u16, "EM Mode"=w284:u8, "Kinetic Series Length"=w286:u16)
        n137 = call "Write JSON.lvclass.vi"("error in (no error)"=w297, "JSON.lvclass"=w298, "Interface in"=w305) -> ("error out"=w301:errorcluster, "Interface out"=w302:refnum<class "Interface.lvclass">)  [unwired: 7 in]
        n138 = local write "Exposure Time"(w295) -> ()
        n139 = local write "Readout Rate"(w294) -> ()
        n140 = local write "Pre-amp gain"(w293) -> ()
        n141 = local write "Initial Line"(w292) -> ()
        n142 = local write "Final Line"(w291) -> ()
        n143 = local write "Final Column"(w290) -> ()
        n144 = local write "Initial Cloumn"(w289) -> ()
        n145 = local write "Binning"(w288) -> ()
        n146 = local write "EM Gain"(w287) -> ()
        n147 = local write "EM Mode"(w284) -> ()
        n148 = local write "Kinetic Series Length"(w286) -> ()
        n149 = case shown="1" w284 {
          tunnel: [string[] ["30 MHz", "20 MHz", "10 MHz", "  1 MHz"] string[] ["   1 MHz", "0.1 MHz"]] -> w285
          frame 0, Default {
          }
          frame 1 {
          }
        }
        n150 = property on="Readout Rate" class="Ring (strict)"("Strings []"=w285) -> ()  [unwired: 2 in, 2 out]
      }
      event "Cooler ON/OFF": Value Change {
        n151 = event-data() -> ()  [unwired: 1 in, 3 out]
        n152 = call "Read CCD.lvclass.vi"("error in (no error)"=w323, "Interface in"=w322) -> ("error out"=w318:errorcluster, "CCD.lvclass"=w319:refnum<class "CCD.lvclass">, "Interface out"=w314:refnum<class "Interface.lvclass">)  [unwired: 7 in]
        n153 = call "Read Cooler.lvclass.vi"("error in (no error)"=w318, "CCD in"=w319) -> ("error out"=w309:errorcluster, "Cooler.lvclass"=w312:refnum<class "Cooler.lvclass">, "CCD out"=w315:refnum<class "CCD.lvclass">)  [unwired: 7 in]
        n154 = case shown="1" "Cooler ON/OFF" {
          tunnel: w312 -> [w325 w333]
          tunnel: [w326 w332] -> w311
          tunnel: [w327 w331] -> w310
          tunnel: w309 -> [w328 w330]
          tunnel: [T4."Disabled and Grayed Out" ("Disabled") T4."Enabled" ("Disabled")] -> w308
          frame 0, Default {
            n155 = call "Cooler OFF.vi"("error in (no error)"=w328, "Cooler in"=w325) -> ("error out"=w327:errorcluster, "Cooler out"=w326:refnum<class "Cooler.lvclass">)  [unwired: 8 in]
          }
          frame 1 {
            n156 = call "Cooler ON.vi"("error in (no error)"=w330, "Cooler in"=w333) -> ("error out"=w331:errorcluster, "Cooler out"=w332:refnum<class "Cooler.lvclass">)  [unwired: 8 in]
          }
        }
        n157 = property on="Set temperature" class="DigNum (strict)"("DisabledEnum"=w308) -> ()  [unwired: 2 in, 2 out]
        n158 = call "Write Cooler.lvclass.vi"("error in (no error)"=w310, "Cooler.lvclass"=w311, "CCD in"=w315) -> ("error out"=w316:errorcluster, "CCD out"=w317:refnum<class "CCD.lvclass">)  [unwired: 7 in]
        n159 = call "Write CCD.lvclass.vi"("error in (no error)"=w316, "CCD.lvclass"=w317, "Interface in"=w314) -> ("error out"=w320:errorcluster, "Interface out"=w321:refnum<class "Interface.lvclass">)  [unwired: 7 in]
      }
      event "Sub Image": Value Change {
        n160 = event-data() -> ()  [unwired: 1 in, 1 out]
        n161 = case shown="\"512 x 512\"" "Sub Image" {
          tunnel: [385 257 1 1] -> w337
          tunnel: [640 768 1024 1024] -> w336
          tunnel: [T4."Disabled and Grayed Out" ("Disabled") T4."Disabled and Grayed Out" ("Disabled") T4."Disabled and Grayed Out" ("Disabled") T4."Enabled" ("Disabled")] -> w335
          frame "256 x 256", Default {
          }
          frame "512 x 512" {
          }
          frame "1024 x 1024" {
          }
          frame "Custom" {
          }
        }
        n162 = local write "Initial Line"(w337) -> ()
        n163 = local write "Initial Cloumn"(w337) -> ()
        n164 = local write "Final Line"(w336) -> ()
        n165 = local write "Final Column"(w336) -> ()
        n166 = property on="Final Line" class="DigNum (strict)"("DisabledEnum"=w335) -> ()  [unwired: 2 in, 2 out]
        n167 = property on="Initial Cloumn" class="DigNum (strict)"("DisabledEnum"=w335) -> ()  [unwired: 2 in, 2 out]
        n168 = property on="Initial Line" class="DigNum (strict)"("DisabledEnum"=w335) -> ()  [unwired: 2 in, 2 out]
        n169 = property on="Final Column" class="DigNum (strict)"("DisabledEnum"=w335) -> ()  [unwired: 2 in, 2 out]
      }
      event "Set temperature": Value Change {
        n170 = event-data() -> ()  [unwired: 1 in, 1 out]
        n171 = call "Read CCD.lvclass.vi"("error in (no error)"=w368, "Interface in"=w369) -> ("error out"=w366:errorcluster, "CCD.lvclass"=w367:refnum<class "CCD.lvclass">, "Interface out"=w361:refnum<class "Interface.lvclass">)  [unwired: 7 in]
        n172 = call "Read Cooler.lvclass.vi"("error in (no error)"=w366, "CCD in"=w367) -> ("error out"=w365:errorcluster, "Cooler.lvclass"=w364:refnum<class "Cooler.lvclass">, "CCD out"=w363:refnum<class "CCD.lvclass">)  [unwired: 7 in]
        n173 = call "Verify Cooler.vi"("error in (no error)"=w365, "Cooler in"=w364) -> ("error out"=w355:errorcluster, "coolerStatus"=w357:bool, "Cooler out"=w356:refnum<class "Cooler.lvclass">)  [unwired: 7 in]
        n174 = case shown="True" w357 {
          tunnel: w356 -> [w371 w376]
          tunnel: w355 -> [w370 w375]
          tunnel: [w371 w374] -> w354
          tunnel: [w370 w373] -> w353
          tunnel: "Set temperature" -> [_ w372]
          frame False {
          }
          frame True {
            n175 = call "Set Temperature.vi"("error in (no error)"=w375, "Numeric Control"=w372, "Cooler in"=w376) -> ("error out"=w373:errorcluster, "Cooler out"=w374:refnum<class "Cooler.lvclass">)  [unwired: 7 in]
          }
        }
        n176 = call "Write Cooler.lvclass.vi"("error in (no error)"=w353, "Cooler.lvclass"=w354, "CCD in"=w363) -> ("error out"=w358:errorcluster, "CCD out"=w362:refnum<class "CCD.lvclass">)  [unwired: 7 in]
        n177 = call "Write CCD.lvclass.vi"("error in (no error)"=w358, "CCD.lvclass"=w362, "Interface in"=w361) -> ("error out"=w359:errorcluster, "Interface out"=w360:refnum<class "Interface.lvclass">)  [unwired: 7 in]
      }
    }
    n178 = Wait Until Next ms Multiple(millisecond multiple=u32 5) -> ()  [unwired: 1 out]
  }
  n179 = call "Read CCD.lvclass.vi"("Interface in"=w35) -> ("error out"=w7:errorcluster, "CCD.lvclass"=w33:refnum<class "CCD.lvclass">, "Interface out"=w34:refnum<class "Interface.lvclass">)  [unwired: 8 in]
  n180 = call "Shut down camera.vi"("error in (no error)"=w7, "CCD in"=w33) -> ("CCD out"=w32:refnum<class "CCD.lvclass">)  [unwired: 8 in, 1 out]
  n181 = call "Write CCD.lvclass.vi"("CCD.lvclass"=w32, "Interface in"=w34) -> ("Interface out"=w31:refnum<class "Interface.lvclass">)  [unwired: 8 in, 1 out]
  n182 = flat-sequence {
    tunnel: w31 -> [_]
    frame #0 {
      w382 = u32 14079702
      w383 = u16 2 items=["Auto", "Open", "Closed"] ("Shutter Mode")
      w389 = u16 1024 ("Final Column")
      w390 = u16 1 ("Initial Line")
      w392 = u8 0 items=["Gain 1", "Gain 2"] ("Pre-amp gain")
      w394 = u8 1 items=["Electron Multiplying", "Conventional"] ("EM Mode")
      w395 = u16 0 items=["Cooler OFF", "Cooler ON"] ("Cooler ON/OFF")
      w406 = i16 0 ("Temperature")
      n183 = local write "Exposing"(FALSE ("Exposing")) -> ()
      n184 = local write "Exposições realizadas"(u8 0 ("Exposições realizadas")) -> ()
      n185 = control-ref of="Initialization"() -> (w400:refnum<vi>)
      n186 = local write "Stop Button"(FALSE ("Stop Button")) -> ()
      n187 = local write "Serial Number"(w406) -> ()
      n188 = local write "% Acquired"(w406) -> ()
      n189 = local write "Initialization"(FALSE ("Initialization")) -> ()
      n190 = local write "Temperature"(w406) -> ()
      n191 = Bundle(u32 1985280, u32 1985280) -> (w402:cluster{u32, u32})  [unwired: 1 in]
      n192 = property on="Temperature" class="DigNum (strict)"("NumText.BGColor"=w382) -> ()  [unwired: 2 in, 2 out]
      n193 = property on="Temperature" class="DigNum (strict)"("NumText.BG Color"=w382) -> ()  [unwired: 2 in, 2 out]
      n194 = Build Array(w402) -> (w401:cluster{u32, u32}[])
      n195 = property on="Property Node" class="Bool (strict)"(reference=w400, "Colors [4]"=w401) -> ()  [unwired: 1 in, 2 out]
      n196 = property on="Set temperature" class="DigNum (strict)"("DisabledEnum"=T4."Disabled and Grayed Out" ("Disabled")) -> ()  [unwired: 2 in, 2 out]
      n197 = local write "Exposure Time"(1e-05 ("Exposure Time")) -> ()
      n198 = local write "Cooler ON/OFF"(w395) -> ()
      n199 = local write "Set temperature"(i8 20 ("Temperature ºC")) -> ()
      n200 = local write "EM Mode"(w394) -> ()
      n201 = local write "EM Gain"(u16 2 ("EM Gain")) -> ()
      n202 = local write "Exposições realizadas"(u8 0 ("Exposições realizadas")) -> ()
      n203 = local write "# Images"(u16 1 ("# Images")) -> ()
      n204 = local write "Kinetic Series Length"(u16 1 ("Kinetic Series Length")) -> ()
      n205 = local write "Readout Rate"(0) -> ()
      n206 = property on="Readout Rate" class="Ring (strict)"("Strings []"=string[] ["   1 MHz", "0.1 MHz"]) -> ()  [unwired: 2 in, 2 out]
      n207 = property on="Exposições realizadas" class="Slide (strict)"("Scale.Maximum"=1.0 ("Scale.Range:Maximum")) -> ()  [unwired: 2 in, 2 out]
      n208 = local write "Shutter Mode"(w383) -> ()
      n209 = local write "Pre-amp gain"(w392) -> ()
      n210 = local write "Sub Image"(T3."1024 x 1024" ("Sub Image")) -> ()
      n211 = local write "Initial Line"(w390) -> ()
      n212 = local write "Initial Cloumn"(w390) -> ()
      n213 = local write "Final Column"(w389) -> ()
      n214 = local write "Final Line"(w389) -> ()
      n215 = local write "Binning"(u8 1 ("Binning")) -> ()
      n216 = local write "Image Name"("" ("Image Name")) -> ()
      n217 = local write "JSON File Path"(path "" ("JSON File Path")) -> ()
    }
  }
